vi "AlAs-GaAs superlattice-111215a.vi"() -> ()   [LabVIEW 2011]
panel:
  in  "As_Gas Flow 2":dbl
  in  "Number of \nGrowth Steps":i32=50
  out "step number":i32
  in  "Aluminum Flow":dbl=10.0
  in  "Ga Flow 1":dbl=5.49
  in  "As_Gas Flow":dbl=33.0
  in  "Manifold H2 Flow":dbl=730.0
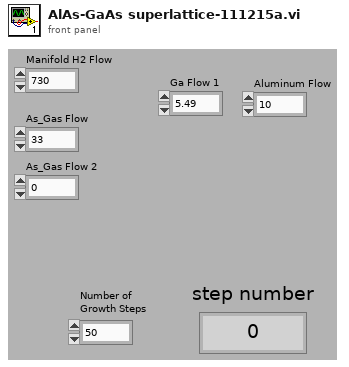
[diagram p1: front panel]
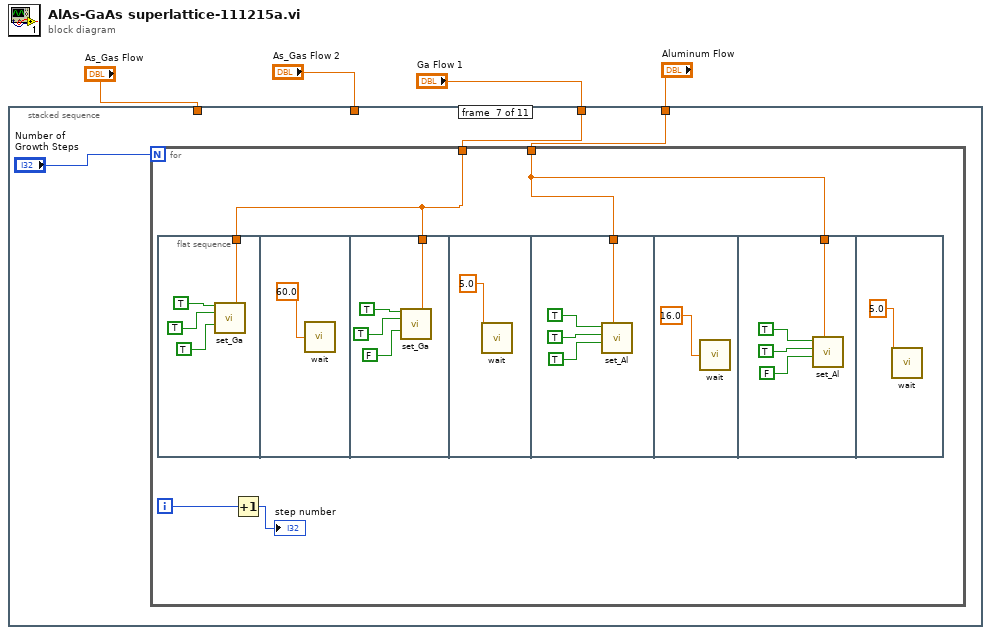
[diagram p0: block diagram]
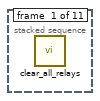
[diagram p2: hidden frame]
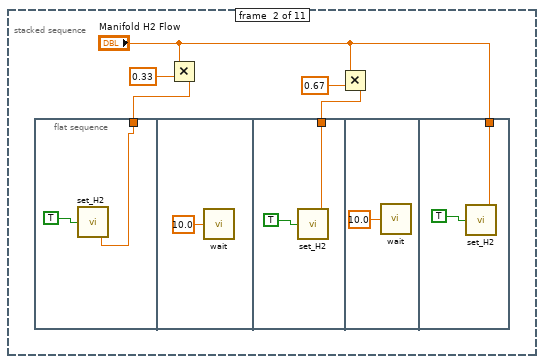
[diagram p3: hidden frame]
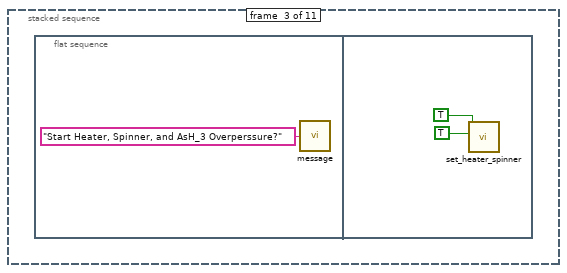
[diagram p4: hidden frame]
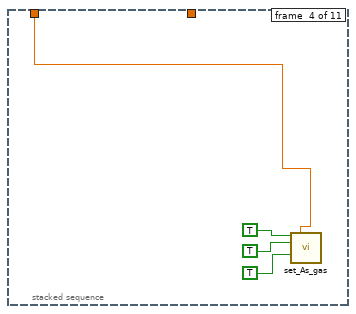
[diagram p5: hidden frame]
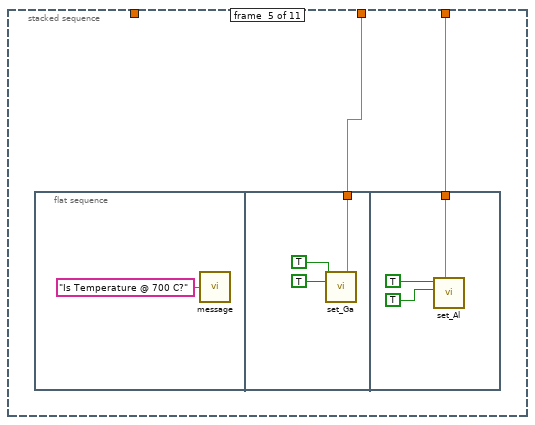
[diagram p6: hidden frame]
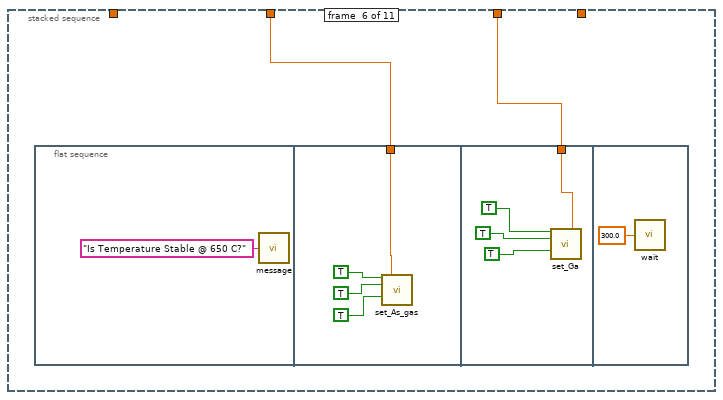
[diagram p7: hidden frame]
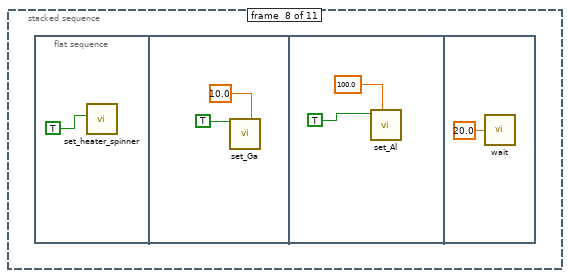
[diagram p8: hidden frame]
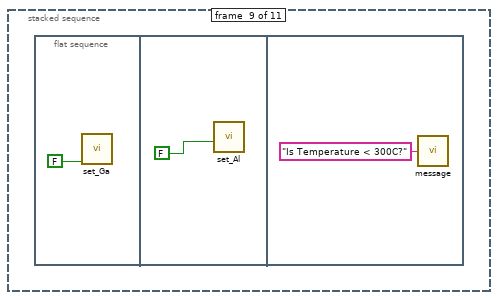
[diagram p9: hidden frame]
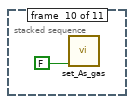
[diagram p10: hidden frame]
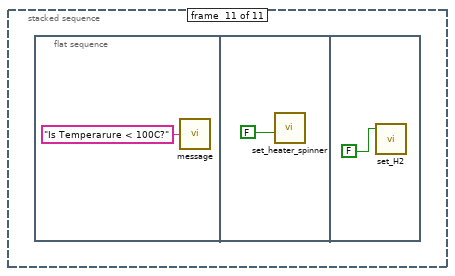
[diagram p11: hidden frame]
diagram:
  n1 = stacked-sequence {
    tunnel: "Ga Flow 1" -> [_ _ _ _ w26 w35 w47 _ _ _ _]
    tunnel: "As_Gas Flow" -> [_ _ _ w21 _ _ _ _ _ _ _]
    tunnel: "Aluminum Flow" -> [_ _ _ _ w25 _ w46 _ _ _ _]
    tunnel: "As_Gas Flow 2" -> [_ _ _ _ _ w34 _ _ _ _ _]
    frame #0 {
      n2 = call "clear_all_relays.vi"() -> ()  [unwired: 2 out]
    }
    frame #1 {
      n3 = flat-sequence {
        tunnel: w9 -> [w10]
        tunnel: w7 -> [w13]
        tunnel: "Manifold H2 Flow" -> [w16]
        frame #0 {
          n4 = call "set_H2.vi"("Manifold H2 Flow"=w10, "H2 Active"=TRUE) -> ()  [unwired: 2 in, 2 out]
        }
        frame #1 {
          n5 = call "wait.vi"("Wait (s)"=10.0) -> ()
        }
        frame #2 {
          n6 = call "set_H2.vi"("Manifold H2 Flow"=w13, "H2 Active"=TRUE) -> ()  [unwired: 2 in, 2 out]
        }
        frame #3 {
          n7 = call "wait.vi"("Wait (s)"=10.0) -> ()
        }
        frame #4 {
          n8 = call "set_H2.vi"("Manifold H2 Flow"=w16, "H2 Active"=TRUE) -> ()  [unwired: 2 in, 2 out]
        }
      }
      n9 = Multiply(x="Manifold H2 Flow", y=0.33) -> (x*y=w9:dbl)
      n10 = Multiply(x="Manifold H2 Flow", y=0.67) -> (x*y=w7:dbl)
    }
    frame #2 {
      n11 = flat-sequence {
        frame #0 {
          n12 = call "message.vi"("message"="Start Heater, Spinner, and AsH_3 Overperssure?") -> ()
        }
        frame #1 {
          n13 = call "set_heater_spinner.vi"("Spinner"=TRUE, "Heater"=TRUE) -> ()  [unwired: 1 in, 7 out]
        }
      }
    }
    frame #3 {
      n14 = call "set_As_gas.vi"("As_Gas Active"=TRUE, "As_Gas Flow"=w21, "As_Gas In"=TRUE, "As_Gas Run"=TRUE) -> ()  [unwired: 2 in, 10 out]
    }
    frame #4 {
      n15 = flat-sequence {
        tunnel: w26 -> [w28]
        tunnel: w25 -> [w31]
        frame #0 {
          n16 = call "message.vi"("message"="Is Temperature @ 700 C?") -> ()
        }
        frame #1 {
          n17 = call "set_Ga.vi"("Ga Active"=TRUE, "Ga Flow 1"=w28, "Ga Bubbler"=TRUE) -> ()  [unwired: 5 in, 8 out]
        }
        frame #2 {
          n18 = call "set_Al.vi"("Aluminum Flow"=w31, "Al Bubbler"=TRUE ("Ga Bubbler"), "Al Active"=TRUE ("Ga Active")) -> ()  [unwired: 2 in, 5 out]
        }
      }
    }
    frame #5 {
      n19 = flat-sequence {
        tunnel: w34 -> [w37]
        tunnel: w35 -> [w41]
        frame #0 {
          n20 = call "message.vi"("message"="Is Temperature Stable @ 650 C?") -> ()
        }
        frame #1 {
          n21 = call "set_As_gas.vi"("As_Gas Active"=TRUE, "As_Gas Flow"=w37, "As_Gas In"=TRUE, "As_Gas Run"=TRUE) -> ()  [unwired: 2 in, 10 out]
        }
        frame #2 {
          n22 = call "set_Ga.vi"("Ga Active"=TRUE ("P_Gas Active"), "Ga Flow 1"=w41, "Ga Bubbler"=TRUE ("P_Gas In"), "Ga Run"=TRUE ("P_Gas Run")) -> ()  [unwired: 4 in, 8 out]
        }
        frame #3 {
          n23 = call "wait.vi"("Wait (s)"=300.0) -> ()
        }
      }
    }
    frame #6 {
      n24 = for {
        N: "Number of \nGrowth Steps" -> [_]
        tunnel: w47 -> [w50]
        tunnel: w46 -> [w49]
        i -> [w51]
        n25 = flat-sequence {
          tunnel: w50 -> [w53]
          tunnel: w50 -> [w58]
          tunnel: w49 -> [w63]
          tunnel: w49 -> [w68]
          frame #0 {
            n26 = call "set_Ga.vi"("Ga Active"=TRUE ("P_Gas Active"), "Ga Flow 1"=w53, "Ga Bubbler"=TRUE ("P_Gas In"), "Ga Run"=TRUE ("P_Gas Run")) -> ()  [unwired: 4 in, 8 out]
          }
          frame #1 {
            n27 = call "wait.vi"("Wait (s)"=60.0) -> ()
          }
          frame #2 {
            n28 = call "set_Ga.vi"("Ga Active"=TRUE ("P_Gas Active"), "Ga Flow 1"=w58, "Ga Bubbler"=TRUE ("P_Gas In"), "Ga Run"=FALSE ("P_Gas Run")) -> ()  [unwired: 4 in, 8 out]
          }
          frame #3 {
            n29 = call "wait.vi"("Wait (s)"=5.0) -> ()
          }
          frame #4 {
            n30 = call "set_Al.vi"("Aluminum Flow"=w63, "Al Run"=TRUE ("P_Gas Run"), "Al Bubbler"=TRUE ("P_Gas In"), "Al Active"=TRUE ("P_Gas Active")) -> ()  [unwired: 1 in, 5 out]
          }
          frame #5 {
            n31 = call "wait.vi"("Wait (s)"=16.0) -> ()
          }
          frame #6 {
            n32 = call "set_Al.vi"("Aluminum Flow"=w68, "Al Run"=FALSE ("P_Gas Run"), "Al Bubbler"=TRUE ("P_Gas In"), "Al Active"=TRUE ("P_Gas Active")) -> ()  [unwired: 1 in, 5 out]
          }
          frame #7 {
            n33 = call "wait.vi"("Wait (s)"=5.0) -> ()
          }
        }
        n34 = Increment(x=w51) -> (x+1=→"step number":i32)
      }
    }
    frame #7 {
      n35 = flat-sequence {
        frame #0 {
          n36 = call "set_heater_spinner.vi"("Spinner"=TRUE ("Ga Active")) -> ()  [unwired: 2 in, 7 out]
        }
        frame #1 {
          n37 = call "set_Ga.vi"("Ga Active"=TRUE, "Ga Flow 1"=10.0) -> ()  [unwired: 6 in, 8 out]
        }
        frame #2 {
          n38 = call "set_Al.vi"("Aluminum Flow"=100.0, "Al Active"=TRUE ("Ga Active")) -> ()  [unwired: 3 in, 5 out]
        }
        frame #3 {
          n39 = call "wait.vi"("Wait (s)"=20.0) -> ()
        }
      }
    }
    frame #8 {
      n40 = flat-sequence {
        frame #0 {
          n41 = call "set_Ga.vi"("Ga Remote"=FALSE) -> ()  [unwired: 7 in, 8 out]
        }
        frame #1 {
          n42 = call "set_Al.vi"("Al Run"=FALSE ("Ga Remote")) -> ()  [unwired: 4 in, 5 out]
        }
        frame #2 {
          n43 = call "message.vi"("message"="Is Temperature < 300C?") -> ()
        }
      }
    }
    frame #9 {
      n44 = call "set_As_gas.vi"("As_Gas Remote"=FALSE) -> ()  [unwired: 5 in, 10 out]
    }
    frame #10 {
      n45 = flat-sequence {
        frame #0 {
          n46 = call "message.vi"("message"="Is Temperarure < 100C?") -> ()
        }
        frame #1 {
          n47 = call "set_heater_spinner.vi"("Heater/Spinner Remote"=FALSE) -> ()  [unwired: 2 in, 7 out]
        }
        frame #2 {
          n48 = call "set_H2.vi"("H2N2 Remote"=FALSE) -> ()  [unwired: 3 in, 2 out]
        }
      }
    }
  }
